vi "SetParameter.vi"(8 "Error In":errorcluster, 10 "Data":variant, 11 "ModuleID":i32) -> (0 "Error Out":errorcluster)   [LabVIEW 2018, in "AcPwrModule.lvlib"]
doc: "This VI sends a message along with the necessary settings to configure the instrument(s). The intended recipient of the message is Main.vi but any VI with a properly set up event structure can listen for this message"
uses:
  AcPwrModule.lvlib
  AcPwrShared/clEventType.ctl
  <vilib>/Utility/error.llb/Error Cluster From Error Code.vi
  <vilib>/ErrorRing/Error Ring.xnode
  AcPwrShared/AcPwrShared.lvlib
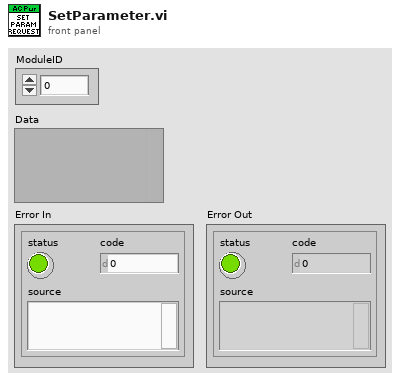
[diagram p1: front panel]
types:
  T1 = typedef "AcPwrShared.lvlib/clRequestEvents.ctl" = cluster{"StopRequest":refnum<user-event>, "PathToINI":refnum<user-event>, " LoadPlugin":refnum<user-event>, "ShowPanel":refnum<user-event>, "PrefDlg":refnum<user-event>, "InitAcPwr":refnum<user-event>, "Reset":refnum<user-event>, "Close":refnum<user-event>, "StopMeas":refnum<user-event>, "StartMeas":refnum<user-event>, "ConfigDevice":refnum<user-event>, "DeviceOn":refnum<user-event>, "DeviceOff":refnum<user-event>, "GetSettings":refnum<user-event>, "SetSettings":refnum<user-event>, "Abort":refnum<user-event>, "SetParameter":refnum<user-event>, "GetSettingsLV":refnum<user-event>}
  T2 = typedef "AcPwrShared.lvlib/clEventType.ctl" = cluster{"ModuleID":i32, "Data":variant}
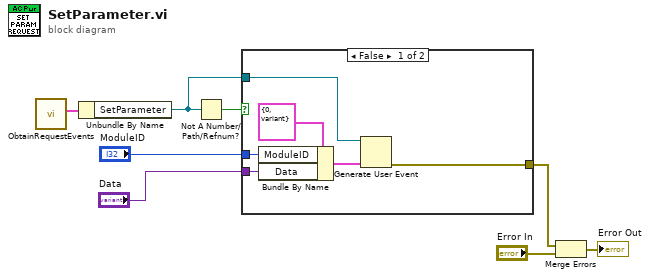
[diagram p0: block diagram]
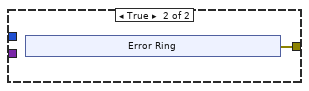
[diagram p2: hidden frame]
diagram:
  n1 = call "ObtainRequestEvents.vi"() -> ("AcPwrRequestEvents"=w8:T1)  [unwired: 10 in, 1 out]
  n2 = Unbundle By Name(w8) -> ("SetParameter"=w2:refnum<user-event>)
  n3 = Not A Number/Path/Refnum?(number/path/refnum=w2) -> (NaN/Path/Refnum?=w7:bool)
  n4 = case shown="False" w7 {
    tunnel: [w14 w15] -> w4
    tunnel: "ModuleID" -> [w12 _]
    tunnel: w2 -> [w10 _]
    tunnel: "Data" -> [w9 _]
    frame False {
      n5 = Bundle By Name(cluster=T2 {"ModuleID"=0, "Data"=variant} ("clEventType"), "ModuleID"=w12, "Data"=w9) -> (w13:T2)
      n6 = Generate User Event(user event=w10, event data cluster=w13) -> (error out=w14:errorcluster)  [unwired: 2 in, 1 out]
    }
    frame True {
      n7 = xnode "Error Ring"() -> ("error out"=w15:errorcluster)
    }
  }
  n8 = Merge Errors(w4, "Error In") -> (→"Error Out":errorcluster)
